vi "Teleop.vi"(10 "Match Info":T2={"Autonomous Elapsed Seconds"=0.0, "TeleOp Elapsed Seconds"=0.0, "Disabled Elapsed Seconds"=0.0, "Visited Autonomous"=FALSE, "Visited TeleOp"=FALSE, "Visited Disabled"=FALSE, "Autonomous Settings"={"Autonomous Style"=enum."Independent", "VI Refnum"=refnum}}, 11 "Call Context":T3) -> ()   [LabVIEW 2016]
doc: "This VI is called for each TeleOp packet received from the DS where the robot is not disabled. It is often used to read from the joysticks and update I/O or to update setpoints for timed control loops. It should complete and return within 20 milliseconds or it may miss DS packets."
uses:
  <vilib>/Rock Robotics/WPI/DriverStation/WPI_DriverStationDerivedRobotMode.ctl
  <vilib>/Rock Robotics/WPI/DriverStation/WPI_DriverStationMatch Info.ctl
  <vilib>/Rock Robotics/WPI/Utilities/WPI_GetSetVariantRefNum.vi
  Robot Global Data.vi
  <vilib>/Rock Robotics/WPI/Solenoid/Deprecated/WPI_SolenoidSetBool.vi
  <vilib>/addons/control/pid/pid.llb/PID (DBL).vi
  navX Library v2/navX Library v2.lvlib
  <vilib>/addons/control/pid/NI_PID_pid.lvlib
panel:
  in  "Mode":bool
  in  "output range":cluster{"output high":dbl, "output low":dbl}={"output high"=100.0, "output low"=-100.0} {"output low" format="%.2f"; "output high" format="%.2f"}
  in  "PID gains":T1={"proportional gain (Kc)"=1.0, "integral time (Ti, min)"=0.01, "derivative time (Td, min)"=0.0} {"derivative time (Td, min)" format="%.3f"; "integral time (Ti, min)" format="%.3f"; "proportional gain (Kc)" format="%.3f"}
  out "Left":dbl(graph)
  out "Right":dbl(graph)
  out "Encoder Right":dbl(graph)
  out "Encoder Left":dbl(graph)
  in  "Speed":dbl=0.5 format="%#_13g"
  out "Out Left":dbl(graph)
  out "Out Right":dbl(graph)
  out "Shooter":cluster{"Sensor Velocity":dbl, dbl, dbl}(graph)
  in  "ShooterRPM":dbl
  in  "P":dbl=0.5 format="%#_13g"
  in  "I":dbl format="%#_13g"
  in  "D":dbl format="%#_13g"
  in  "F":dbl=0.005212 format="%#_13g"
  in  "I Zone":dbl format="%#_13g"
  in  "Ramp Rate":dbl format="%#_13g"
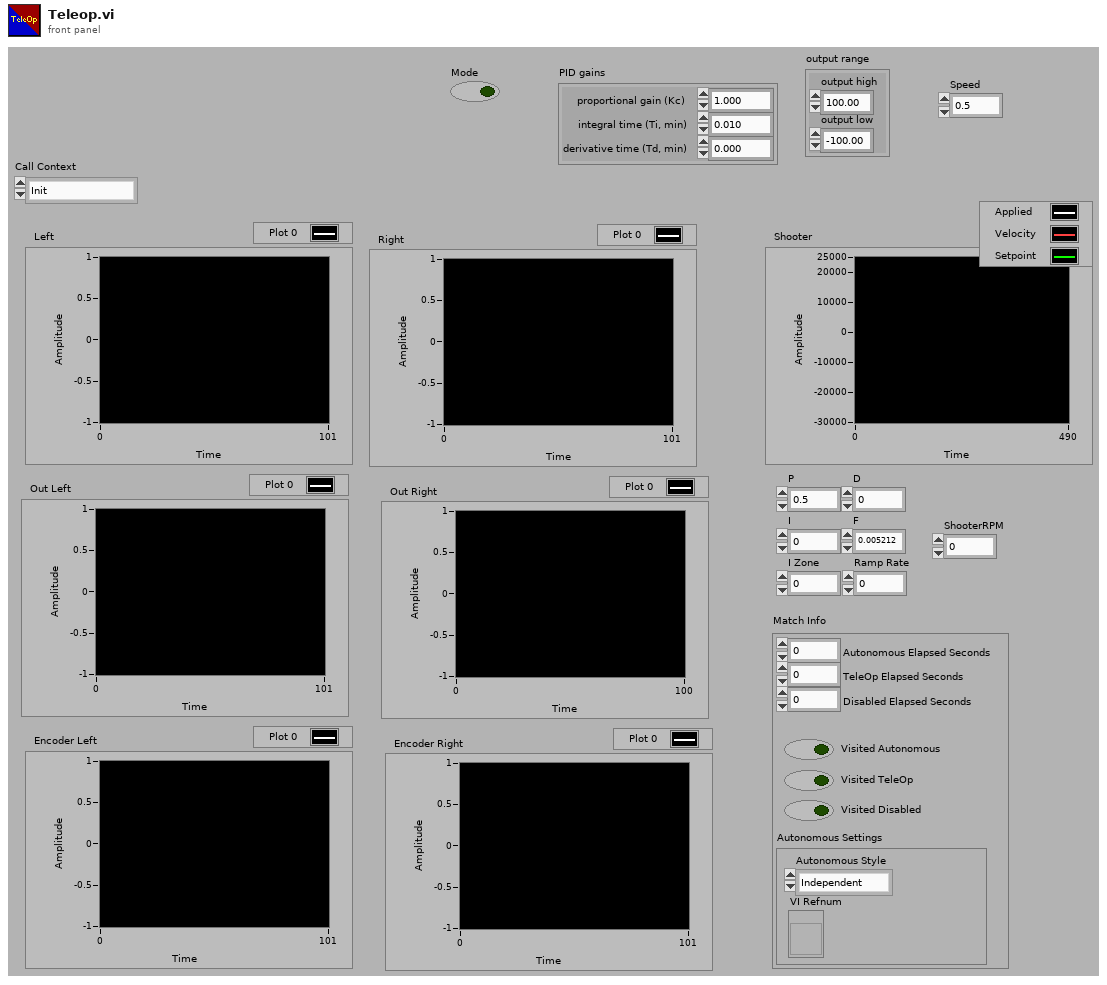
[diagram p1: front panel]
types:
  T1 = cluster{"proportional gain (Kc)":dbl, "integral time (Ti, min)":dbl, "derivative time (Td, min)":dbl}
  T2 = typedef "WPI_DriverStationMatch Info.ctl" = cluster{"Autonomous Elapsed Seconds":dbl, "TeleOp Elapsed Seconds":dbl, "Disabled Elapsed Seconds":dbl, "Visited Autonomous":bool, "Visited TeleOp":bool, "Visited Disabled":bool, "Autonomous Settings":cluster{"Autonomous Style":enum16{"Iterative", "Independent"}, "VI Refnum":refnum<vi>}}
  T3 = typedef "WPI_DriverStationDerivedRobotMode.ctl" = enum16{"Init", "Execute", "Stop"}
  T4 = typedef "WPI_SolenoidDevRef.ctl" = cluster{"DevStatus":errorcluster, "Pneumatics Control Module":u8, "Forward Solenoid Channel":T5, "Reverse Solenoid Channel":T5}
  T5 = typedef "WPI_SolenoidChannel.ctl" = enum8{"Solenoid 0", "Solenoid 1", "Solenoid 2", "Solenoid 3", "Solenoid 4", "Solenoid 5", "Solenoid 6", "Solenoid 7", "Invalid"}
  T6 = typedef "WPI_JoystickDevRef.ctl" = cluster{"Device":T7}
  T7 = typedef "WPI_JoystickDeviceEnum.ctl" = enum16{"USB 0", "USB 1", "USB 2", "USB 3", "USB 4", "USB 5"}
  T8 = cluster{"Buttons[0]":bool, "Buttons[1]":bool, "Buttons[2]":bool, "Buttons[3]":bool, "Buttons[4]":bool, "Buttons[5]":bool, "Buttons[6]":bool, "Buttons[7]":bool, "Buttons[8]":bool}
  T9 = cluster{"Axes[0]":dbl, "Axes[1]":dbl, "Axes[2]":dbl, "Axes[3]":dbl, "Axes[4]":dbl, "Axes[5]":dbl, "Axes[6]":dbl, "Axes[7]":dbl, "Axes[8]":dbl}
  T10 = typedef "navX Library v2.lvlib/Z900_navX_DeviceTypeDef.ctl" = cluster{"Interface":cluster{"Protocol":T11, "Update Rate (4Hz-100Hz)":u8, "navX Open TypeDef":variant}, "Notify Packet":refnum<notifier>, "Loop VI Refnum":refnum<vi>, "Ready to Close Occurrence Refnum":refnum<k4>}
  T11 = typedef "navX Library v2.lvlib/Z900_navX_ProtocolTypeDef.ctl" = enum16{"SERIAL", "I2C", "SPI"}
  T12 = cluster{"Velocity X":dbl, "Velocity Y":dbl, "Velocity Z":dbl, "Displacement X":dbl, "Displacement Y":dbl, "Displacement Z":dbl}
  T13 = cluster{"LinearAcceleration X":dbl, "LinearAcceleration Y":dbl, "LinearAcceleration Z":dbl}
  T14 = cluster{"Quat W":dbl, "Quat X":dbl, "Quat Y":dbl, "Quat Z":dbl}
  T15 = cluster{"Yaw":dbl, "Roll":dbl, "Pitch":dbl, "Heading":dbl, "Fused Heading":dbl}
  T16 = cluster{"Velocity X":dbl, "Velocity Y":dbl, "Velocity Z":dbl, "Displacement X":dbl, "Displacement Y":dbl, "Displacement Z":dbl, "LinearAcceleration X":dbl, "LinearAcceleration Y":dbl, "LinearAcceleration Z":dbl, "Quat W":dbl, "Quat X":dbl, "Quat Y":dbl, "Quat Z":dbl, "Yaw":dbl, "Roll":dbl, "Pitch":dbl}
  T17 = typedef "WPI_MotorControlDeviceRef.ctl" = cluster{"DeviceStatus":errorcluster, "Type":T18, "PWM":cluster{"PWM Channel":T19, "DeadBand":T20}, "CAN":cluster{"Device Number":u8, "SetOutput VI Ref":variant, "GetOutput VI Ref":variant, "Enable VI Ref":variant, "Disable VI Ref":variant, "Data":variant}, "Invert":bool}
  T18 = typedef "WPI_MotorControlType.ctl" = enum16{"PWM", "CAN"}
  T19 = typedef "FPGA_DIOPWMChannel.ctl" = enum8{"PWM 0", "PWM 1", "PWM 2", "PWM 3", "PWM 4", "PWM 5", "PWM 6", "PWM 7", "PWM 8", "PWM 9", "PWM MXP 0", "PWM MXP 1", "PWM MXP 2", "PWM MXP 3", "PWM MXP 4", "PWM MXP 5", "PWM MXP 6", "PWM MXP 7", "PWM MXP 8", "PWM MXP 9", "Invalid"}
  T20 = typedef "WPI_PWMDeadband.ctl" = cluster{"Name":string, "maxPositivePwm":i32, "minPositivePwm":i32, "centerPwm":i32, "maxNegativePwm":i32, "minNegativePwm":i32, "angularRange":u16}
  T21 = typedef "WPI_CANTalonSRX_GlobalStatus.ctl" = cluster{"Applied Throttle":dbl, "Module Enabled":bool, "CAN Error":errorcluster, "Closed Loop Error":dbl, "Forward Limit Switch Closed":bool, "Reverse Limit Switch Closed":bool, "Sensor Position":dbl, "Sensor Velocity":dbl, "Current":dbl, "Sticky Fault - Over Temp":bool, "Sticky Fault - Under Voltage":bool, "Sticky Fault - Forward Limit":bool, "Sticky Fault - Reverse Limit":bool, "Sticky Fault - Forward Soft Limit":bool, "Sticky Fault - Reverse Soft Limit":bool, "Brake is Enabled":bool, "Encoder Position":dbl, "Encoder Velocity":dbl, "Encoder Index Count":dbl, "Encoder A Pin State":bool, "Encoder B Pin State":bool, "Encoder Index Pin State":bool, "Analog In":dbl, "Analog In Velocity":dbl, "Temperature (C)":dbl, "Battery Voltage":dbl, "Control 5 Is Supported":bool, "Current Profile Slot Select":dbl, "Pos Div 8":bool, "Vel Div 4":bool, "Pulse Width Position":i32, "Pulse Width Velocity":i32, "Pulse Width Rise To Rise (us)":i32, "Pulse Width Rise To Fall (us)":i32, "Mot Prof Active Is Under Run":bool, "Mot Prof Active Has Under Run":bool, "Mot Prof Active Is Last":bool, "Mot Prof Active Velocity Only":bool, "Mot Prof Active Is Valid":bool, "Mot Prof Buffer Is Full":bool, "Mot Prof Active Profile Slot Select":i32, "Mot Prof NextID":i32, "Mot Prof Count":i32, "Mot Prof Active Velocity":dbl, "Mot Prof Active Position":dbl, "Mot Prof Output Enable":i32}
  T22 = cluster{dbl, "Sensor Velocity":dbl, "ShooterRPM":dbl}
  T23 = typedef "WPI_RobotDriveDevRef.ctl" = cluster{"DevStatus":errorcluster, "Motors[]":T17[], "Square Inputs":bool, "Max Output":dbl}
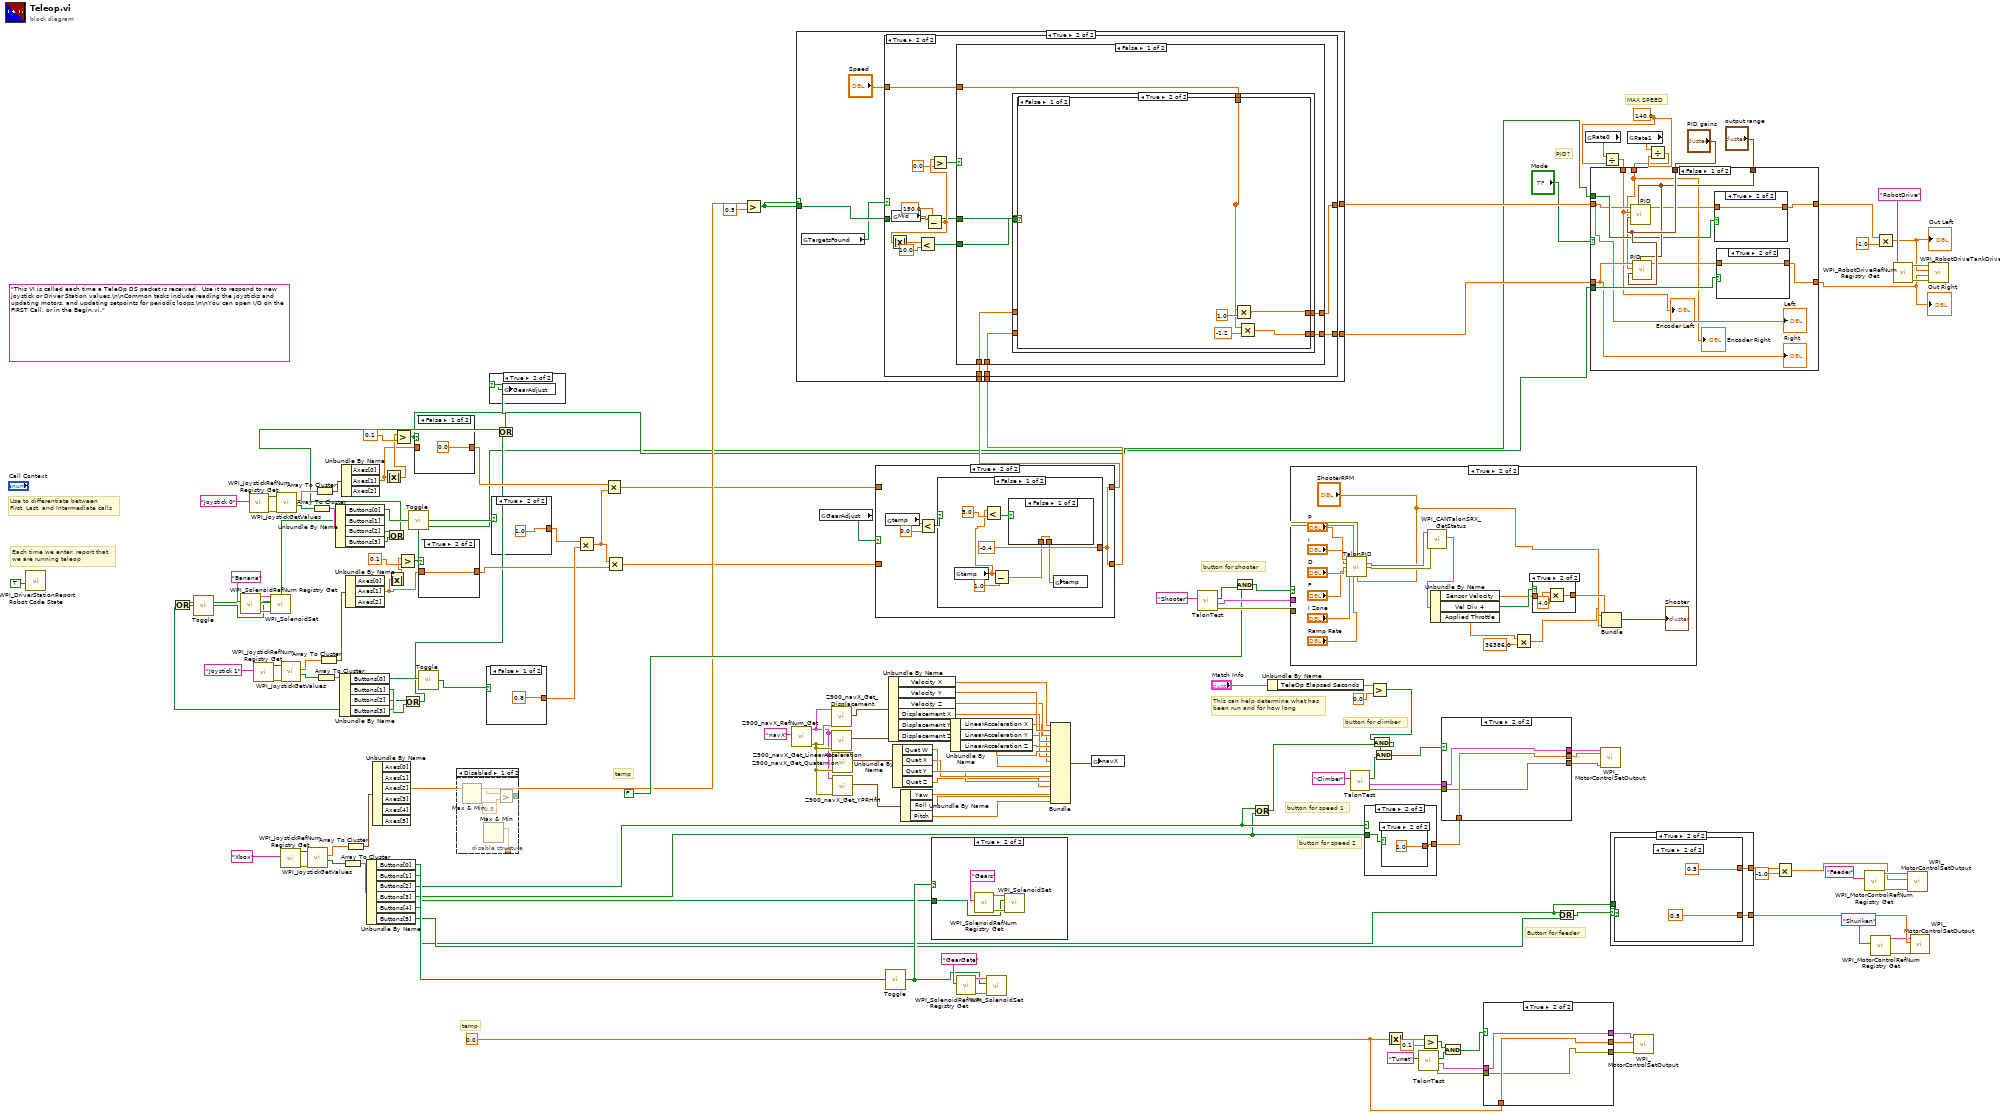
[diagram p0: block diagram]
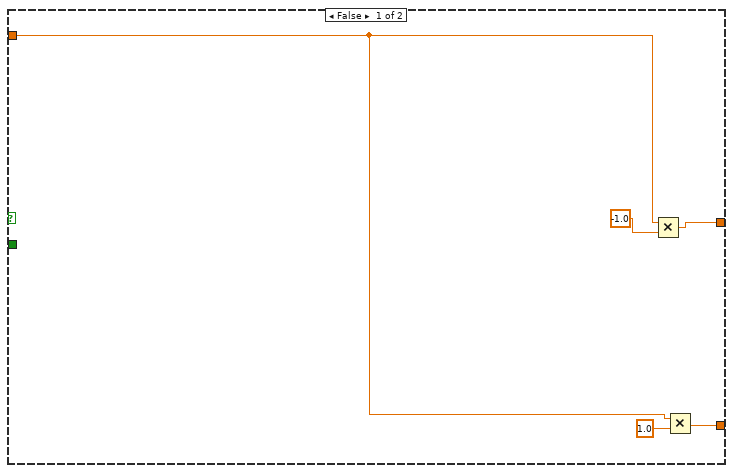
[diagram p3: hidden frame]
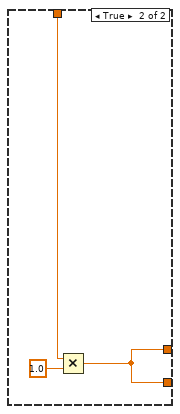
[diagram p5: hidden frame]
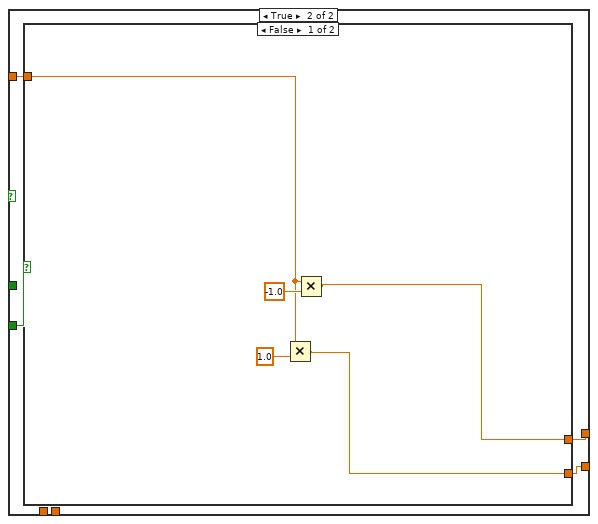
[diagram p6: hidden frame]
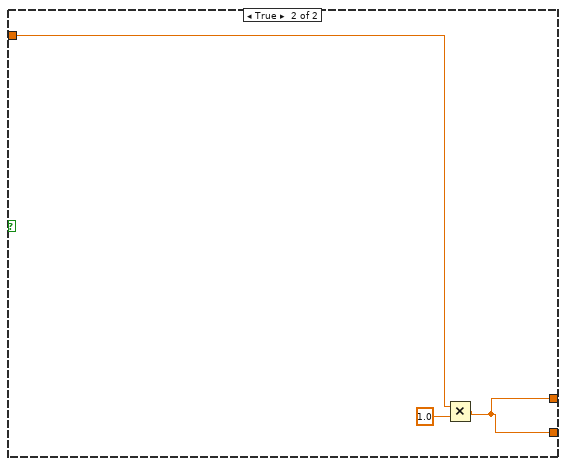
[diagram p7: hidden frame]
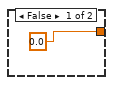
[diagram p8: hidden frame]
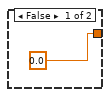
[diagram p9: hidden frame]
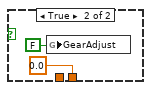
[diagram p14: hidden frame]
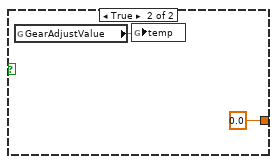
[diagram p15: hidden frame]
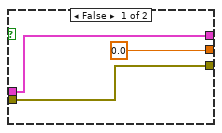
[diagram p16: hidden frame]
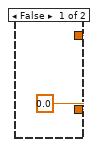
[diagram p18: hidden frame]
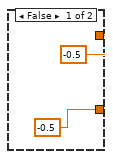
[diagram p19: hidden frame]
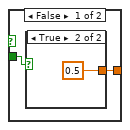
[diagram p20: hidden frame]
diagram:
  w15 = 140.0
  w28 = 0.0
  (unwired) "This VI is called each time a TeleOp DS packet is received.  Use it to respond to new joystick or Driver Station values.\n\nCommon tasks include reading the joysticks and updating motors, and updating setpoints for periodic loops.\n\nYou can open I/O on the FIRST Call, or in the Begin.vi."
  # "MAX SPEED"
  # "PID?"
  # "temp"
  # "temp"
  # "Button for feeder"
  # "button for speed 2"
  # "button for speed 1"
  # "button for climber"
  # "button for shooter"
  # "Each time we enter, report that\nwe are running teleop"
  # "Use to differentiate between\nFirst, Last, and Intermediate calls"
  # "This can help determine what has\nbeen run and for how long"
  n1 = call <vilib>:"WPI_DriverStationReport Robot Code State.vi"("TeleOp"=TRUE ("Autonomous")) -> ()  [unwired: 10 in, 1 out]
  n2 = call <vilib>:"WPI_SolenoidRefNum Registry Get.vi"("refnum name"="Banana") -> ("error out"=w53:errorcluster, "SolenoidDevRef"=w52:T4)  [unwired: 9 in]
  n3 = call <vilib>:"WPI_JoystickRefNum Registry Get.vi"("refnum name"="Joystick 0") -> ("error out"=w155:errorcluster, "JoystickDevRef"=w154:T6)  [unwired: 9 in]
  n4 = call <vilib>:"WPI_JoystickRefNum Registry Get.vi"("refnum name"="Joystick 1") -> ("error out"=w147:errorcluster, "JoystickDevRef"=w146:T6)  [unwired: 9 in]
  n5 = call <vilib>:"WPI_JoystickGetValues.vi"("error in (no error)"=w155, "JoystickDevRef"=w154) -> ("Buttons"=w151:bool[], "Axes"=w152:dbl[])  [unwired: 5 in, 3 out]
  n6 = call <vilib>:"WPI_JoystickRefNum Registry Get.vi"("refnum name"="Xbox") -> ("error out"=w82:errorcluster, "JoystickDevRef"=w81:T6)  [unwired: 9 in]
  n7 = call <vilib>:"WPI_JoystickGetValues.vi"("error in (no error)"=w147, "JoystickDevRef"=w146) -> ("Buttons"=w143:bool[], "Axes"=w144:dbl[])  [unwired: 5 in, 3 out]
  n8 = call <vilib>:"WPI_JoystickGetValues.vi"("error in (no error)"=w82, "JoystickDevRef"=w81) -> ("Buttons"=w78:bool[], "Axes"=w79:dbl[])  [unwired: 5 in, 3 out]
  n9 = Array To Cluster(array=w151) -> (cluster=w149:T8)
  n10 = Array To Cluster(array=w152) -> (cluster=w150:T9)
  n11 = Array To Cluster(array=w143) -> (cluster=w141:T8)
  n12 = Array To Cluster(array=w144) -> (cluster=w142:T9)
  n13 = Unbundle By Name(w149) -> ("Buttons[0]"=w135:bool, "Buttons[1]"=w49:bool, "Buttons[2]"=w34:bool, "Buttons[3]"=w33:bool)
  n14 = Unbundle By Name(w141) -> ("Buttons[0]"=w134:bool, "Buttons[1]"=w48:bool, "Buttons[2]"=w36:bool, "Buttons[3]"=w35:bool)
  n15 = Or(x=w49, y=w48) -> (x .or. y?=w50:bool)
  n16 = call "Toggle.vi"("Input"=w50) -> ("Output"=w47:bool)
  n17 = call-poly <vilib>:"WPI_SolenoidSet.vi"("error in (no error)"=w53, "Value"=w47, "SolenoidDevRef"=w52) -> ()  [unwired: 7 in, 2 out]
  n18 = Unbundle By Name(w150) -> ("Axes[1]"=w136:dbl)  [unwired: 2 out]
  n19 = Array To Cluster(array=w78) -> (cluster=w76:T8)
  n20 = Unbundle By Name(w142) -> ("Axes[1]"=w138:dbl)  [unwired: 2 out]
  n21 = Array To Cluster(array=w79) -> (cluster=w77:T9)
  n22 = Unbundle By Name(w76) -> ("Buttons[0]"=w75:bool, "Buttons[1]"=w74:bool, "Buttons[2]"=w73:bool, "Buttons[3]"=w72:bool, "Buttons[4]"=w69:bool, "Buttons[5]"=w70:bool)
  n23 = Unbundle By Name(w77) -> ("Axes[2]"=w26:dbl)  [unwired: 5 out]
  n24 = Absolute Value(x=w136) -> (abs(x)=w137:dbl)
  n25 = Or(x=w34, y=w33) -> (x .or. y?=w32:bool)
  n26 = Absolute Value(x=w138) -> (abs(x)=w139:dbl)
  n27 = Greater?(x=w137, y=0.1 ("x")) -> (0:w5:bool)
  n28 = Greater?(x=w139, y=0.1 ("x")) -> (0:w4:bool)
  n29 = Or(x=w36, y=w35) -> (x .or. y?=w31:bool)
  n30 = call "Toggle.vi"("Input"=w135) -> ("Output"=w133:bool)
  n31 = case shown="False" w5 {
    tunnel: w136 -> [_ w158]
    tunnel: [0.0 w158] -> w128
    frame False {
    }
    frame True {
    }
  }
  n32 = case shown="True" w4 {
    tunnel: w138 -> [_ w160]
    tunnel: [0.0 w160] -> w129
    frame False {
    }
    frame True {
    }
  }
  n33 = call "Toggle.vi"("Input"=w134) -> ("Output"=w132:bool)
  n34 = disable-structure shown="Disabled" {
    disable-tunnel: [w162 _] -> _
    disable-tunnel: [w161 _] -> _
    frame Disabled {
      n35 = Max & Min() -> (max(x,y)=w164:dbl)  [unwired: 2 in, 1 out]
      n36 = Max & Min() -> (max(x,y)=w161:dbl)  [unwired: 2 in, 1 out]
      n37 = Greater?(x=w164, y=0.5) -> (0:w162:bool)
    }
    frame Enabled {
    }
  }
  n38 = case shown="False" w132 {
    tunnel: [0.8 1.0] -> w130
    frame False {
    }
    frame True {
    }
  }
  n39 = case shown="True" w133 {
    tunnel: [-1.0 1.0] -> w131
    frame False {
    }
    frame True {
    }
  }
  n40 = Or(x=w32, y=w31) -> (x .or. y?=w29:bool)
  n41 = case shown="True" w29 {
    selector: w29 -> [_ w169]
    frame False {
    }
    frame True {
      n42 = global write "Robot Global Data.vi" "GearAdjust"(w169) -> ()
    }
  }
  n43 = Multiply(x=w131, y=w130) -> (x*y=w127:dbl)
  n44 = Multiply(x=w128, y=w127) -> (x*y=w3:dbl)
  n45 = Multiply(x=w127, y=w129) -> (x*y=w2:dbl)
  n46 = Greater?(x=w26, y=0.5) -> (0:w1:bool)
  n47 = call "Z900_navX_RefNum_Get.vi"("refnum name"="navX") -> ("error out"=w125:errorcluster, "navX Device"=w124:T10)  [unwired: 9 in]
  n48 = global read "Robot Global Data.vi" "GearAdjust"() -> (w30:bool)
  n49 = call "Z900_navX_Get_Displacement.vi"("error in (no error)"=w125, "navX Device"=w124) -> ("Displacement"=w120:T12)  [unwired: 6 in, 3 out]
  n50 = call "Z900_navX_Get_LinearAcceleration.vi"("error in (no error)"=w125, "navX Device"=w124) -> ("Linear Acceleration"=w121:T13)  [unwired: 6 in, 3 out]
  n51 = call "Z900_navX_Get_Quaternion.vi"("error in (no error)"=w125, "navX Device"=w124) -> ("Quaternion"=w122:T14)  [unwired: 6 in, 3 out]
  n52 = call "Z900_navX_Get_YPRHfH.vi"("error in (no error)"=w125, "navX Device"=w124) -> ("YRPHfH"=w123:T15)  [unwired: 6 in, 3 out]
  n53 = case shown="True" w30 {
    tunnel: w3 -> [w171 _]
    tunnel: w2 -> [w170 _]
    tunnel: [w171 w172] -> w21
    tunnel: [w170 w172] -> w20
    frame False {
    }
    frame True {
      n54 = global read "Robot Global Data.vi" "temp"() -> (w175:dbl)
      n55 = Less?(x=w175, y=0.0) -> (x < y?=w173:bool)
      n56 = case shown="False" w173 {
        tunnel: [-0.4 0.0] -> w172
        frame False {
          n57 = global read "Robot Global Data.vi" "temp"() -> (w178:dbl)
          n58 = Less?(x=w178, y=5.0 ("x")) -> (x < y?=w179:bool)
          n59 = Subtract(x=w178, y=1.0) -> (x-y=w176:dbl)
          n60 = case shown="False" w179 {
            tunnel: [w183 0.0] -> w177
            tunnel: w176 -> [w183 _]
            frame False {
            }
            frame True {
              n61 = global write "Robot Global Data.vi" "GearAdjust"(FALSE) -> ()
            }
          }
          n62 = global write "Robot Global Data.vi" "temp"(w177) -> ()
        }
        frame True {
          n63 = global read "Robot Global Data.vi" "GearAdjustValue"() -> (w187:dbl)
          n64 = global write "Robot Global Data.vi" "temp"(w187) -> ()
        }
      }
    }
  }
  n65 = case shown="True" w1 {
    tunnel: w21 -> [w189 w196]
    tunnel: w20 -> [w188 w195]
    tunnel: w1 -> [_ w193]
    tunnel: [w189 w192] -> w11
    tunnel: [w188 w191] -> w10
    frame False {
    }
    frame True {
      n66 = global read "Robot Global Data.vi" "TargetsFound"() -> (w190:bool)
      n67 = case shown="True" w190 {
        tunnel: w196 -> [_ w210]
        tunnel: w195 -> [_ w209]
        tunnel: [w199 w208] -> w191
        tunnel: [w200 w207] -> w192
        tunnel: w193 -> [_ w203]
        tunnel: "Speed" -> [w197 w202]
        frame False {
          n68 = Multiply(x=w197, y=-1.0) -> (x*y=w200:dbl)
          n69 = Multiply(x=w197, y=1.0) -> (x*y=w199:dbl)
        }
        frame True {
          n70 = global read "Robot Global Data.vi" "Mid"() -> (w215:dbl)
          n71 = Subtract(x=w215, y=150.0) -> (x-y=w205:dbl)
          n72 = Absolute Value(x=w205) -> (abs(x)=w213:dbl)
          n73 = Less?(x=w213, y=10.0) -> (x < y?=w211:bool)
          n74 = Greater?(x=w205, y=0.0) -> (0:w206:bool)
          n75 = case shown="False" w206 {
            tunnel: w211 -> [w222 w240]
            tunnel: w210 -> [w221 _]
            tunnel: w209 -> [w220 _]
            tunnel: [w219 w238] -> w208
            tunnel: [w218 w239] -> w207
            tunnel: w203 -> [w217 _]
            tunnel: w202 -> [w216 w237]
            frame False {
              n76 = case shown="True" w217 {
                tunnel: w222 -> [_ w228]
                tunnel: w221 -> [w224 _]
                tunnel: w220 -> [w223 _]
                tunnel: [w224 w227] -> w218
                tunnel: [w223 w226] -> w219
                tunnel: w216 -> [_ w225]
                frame False {
                }
                frame True {
                  n77 = case shown="False" w228 {
                    tunnel: [w233 w236] -> w227
                    tunnel: [w231 w236] -> w226
                    tunnel: w225 -> [w229 w234]
                    frame False {
                      n78 = Multiply(x=w229, y=1.0) -> (x*y=w233:dbl)
                      n79 = Multiply(x=w229, y=-1.2) -> (x*y=w231:dbl)
                    }
                    frame True {
                      n80 = Multiply(x=w234, y=1.0) -> (x*y=w236:dbl)
                    }
                  }
                }
              }
            }
            frame True {
              n81 = case shown="False" w240 {
                tunnel: [w245 w248] -> w239
                tunnel: [w243 w248] -> w238
                tunnel: w237 -> [w241 w246]
                frame False {
                  n82 = Multiply(x=w241, y=1.0) -> (x*y=w243:dbl)
                  n83 = Multiply(x=w241, y=-1.0) -> (x*y=w245:dbl)
                }
                frame True {
                  n84 = Multiply(x=w246, y=1.0) -> (x*y=w248:dbl)
                }
              }
            }
          }
        }
      }
    }
  }
  n85 = call "Toggle.vi"("Input"=w75) -> ("Output"=w83:bool)
  n86 = Unbundle By Name(w120) -> ("Velocity X"=w119:dbl, "Velocity Y"=w118:dbl, "Velocity Z"=w117:dbl, "Displacement X"=w116:dbl, "Displacement Y"=w115:dbl, "Displacement Z"=w114:dbl)
  n87 = Unbundle By Name(w122) -> ("Quat W"=w110:dbl, "Quat X"=w109:dbl, "Quat Y"=w108:dbl, "Quat Z"=w107:dbl)
  n88 = Unbundle By Name(w123) -> ("Yaw"=w106:dbl, "Roll"=w105:dbl, "Pitch"=w104:dbl)
  n89 = case shown="True" w83 {
    tunnel: w74 -> [_ w249]
    frame False {
    }
    frame True {
      n90 = call <vilib>:"WPI_SolenoidRefNum Registry Get.vi"("refnum name"="Gears") -> ("error out"=w252:errorcluster, "SolenoidDevRef"=w251:T4)  [unwired: 9 in]
      n91 = call-poly <vilib>:"WPI_SolenoidSet.vi"("error in (no error)"=w252, "Value"=w249, "SolenoidDevRef"=w251) -> ()  [unwired: 7 in, 2 out]
    }
  }
  n92 = Unbundle By Name(w121) -> ("LinearAcceleration X"=w113:dbl, "LinearAcceleration Y"=w112:dbl, "LinearAcceleration Z"=w111:dbl)
  n93 = call <vilib>:"WPI_SolenoidRefNum Registry Get.vi"("refnum name"="GearGate") -> ("error out"=w86:errorcluster, "SolenoidDevRef"=w85:T4)  [unwired: 9 in]
  n94 = call-poly <vilib>:"WPI_SolenoidSet.vi"("error in (no error)"=w86, "Value"=w83, "SolenoidDevRef"=w85) -> ()  [unwired: 7 in, 2 out]
  n95 = Bundle("Velocity X"=w119, "Velocity Y"=w118, "Velocity Z"=w117, "Displacement X"=w116, "Displacement Y"=w115, "Displacement Z"=w114, "LinearAcceleration X"=w113, "LinearAcceleration Y"=w112, "LinearAcceleration Z"=w111, "Quat W"=w110, "Quat X"=w109, "Quat Y"=w108, "Quat Z"=w107, "Yaw"=w106, "Roll"=w105, "Pitch"=w104) -> (w103:T16)  [unwired: 1 in]
  n96 = global write "Robot Global Data.vi" "navX"(w103) -> ()
  n97 = call "TalonTest.vi"("Name"="Shooter") -> ("Output"=w97:bool, "Ref"=w101:T17, "error out"=w100:errorcluster)  [unwired: 7 in]
  n98 = And(x=FALSE, y=w97) -> (x .and. y?=w98:bool)
  n99 = Or(x=w73, y=w72) -> (x .or. y?=w71:bool)
  n100 = Unbundle By Name("Match Info") -> ("TeleOp Elapsed Seconds"=w93:dbl)
  n101 = case shown="True" w98 {
    tunnel: w101 -> [_ w257]
    tunnel: w100 -> [_ w256]
    frame False {
    }
    frame True {
      n102 = call "TalonPID.vi"("P"="P", "Ref In"=w257, "Error in"=w256, "I"="I", "D"="D", "F"="F", "I Zone"="I Zone", "Ramp Rate"="Ramp Rate", "Output"="ShooterRPM") -> ("Ref Out"=w255:T17, "error out"=w254:errorcluster)  [unwired: 5 in]
      n103 = call <vilib>:"WPI_CANTalonSRX_GetStatus.vi"("error in (no error)"=w254, "CAN Talon SRX Ref"=w255) -> ("Talon SRX Status"=w271:T21)  [unwired: 7 in, 2 out]
      n104 = Unbundle By Name(w271) -> ("Sensor Velocity"=w269:dbl, "Vel Div 4"=w270:bool, "Applied Throttle"=w266:dbl)
      n105 = Multiply(x=w266, y=36386.0) -> (x*y=w265:dbl)
      n106 = case shown="True" w270 {
        tunnel: w269 -> [w272 w274]
        tunnel: [w272 w275] -> w264
        frame False {
        }
        frame True {
          n107 = Multiply(x=w274, y=4.0) -> (x*y=w275:dbl)
        }
      }
      n108 = Bundle(w265, "Sensor Velocity"=w264, "ShooterRPM"="ShooterRPM") -> (→"Shooter":T22)  [unwired: 1 in]
    }
  }
  n109 = call "TalonTest.vi"("Name"="Climber") -> ("Output"=w95:bool, "Ref"=w89:T17, "error out"=w88:errorcluster)  [unwired: 7 in]
  n110 = case shown="True" w73 {
    tunnel: [w277 w281] -> w87
    tunnel: w72 -> [w276 w280]
    frame False {
      n111 = case shown="True" w276 {
        tunnel: [0.0 0.5] -> w277
        frame False {
        }
        frame True {
        }
      }
    }
    frame True {
      n112 = case shown="True" w280 {
        tunnel: [0.75 1.0] -> w281
        frame False {
        }
        frame True {
        }
      }
    }
  }
  n113 = Greater?(x=w93, y=0.0) -> (0:w91:bool)
  n114 = And(x=w91, y=w71) -> (x .and. y?=w96:bool)
  n115 = And(x=w96, y=w95) -> (x .and. y?=w90:bool)
  n116 = Absolute Value(x=w28) -> (abs(x)=w62:dbl)
  n117 = call "TalonTest.vi"("Name"="Turret") -> ("Output"=w66:bool, "Ref"=w64:T17, "error out"=w63:errorcluster)  [unwired: 7 in]
  n118 = Greater?(x=w62, y=0.1) -> (0:w60:bool)
  n119 = case shown="True" w90 {
    tunnel: w89 -> [w285 w289]
    tunnel: w88 -> [w284 w287]
    tunnel: w87 -> [_ w288]
    tunnel: [w285 w289] -> w55
    tunnel: [0.0 w288] -> w56
    tunnel: [w284 w287] -> w54
    frame False {
    }
    frame True {
    }
  }
  n120 = And(x=w60, y=w66) -> (x .and. y?=w65:bool)
  n121 = case shown="True" w65 {
    tunnel: w64 -> [w291 w295]
    tunnel: w63 -> [w290 w293]
    tunnel: w28 -> [_ w294]
    tunnel: [w291 w295] -> w59
    tunnel: [0.0 w294] -> w58
    tunnel: [w290 w293] -> w57
    frame False {
    }
    frame True {
    }
  }
  n122 = Or(x=w69, y=w70) -> (x .or. y?=w68:bool)
  n123 = global read "Robot Global Data.vi" "Rate0"() -> (w17:dbl)
  n124 = call <vilib>:"WPI_MotorControlSetOutput.vi"("error in (no error)"=w54, "Output"=w56, "MotorControlDevRef"=w55) -> ()  [unwired: 6 in, 3 out]
  n125 = Divide(x=w17, y=w15) -> (x/y=w14:dbl)
  n126 = case shown="True" w68 {
    tunnel: w69 -> [_ w299]
    tunnel: [w296 w298] -> w39
    tunnel: [w296 w297] -> w46
    frame False {
      w296 = 0.0
    }
    frame True {
      n127 = case shown="True" w299 {
        tunnel: [-0.5 ("Output") 0.5 ("Output")] -> w298
        tunnel: [-0.5 ("Output") 0.5 ("Output")] -> w297
        frame False {
        }
        frame True {
        }
      }
    }
  }
  n128 = global read "Robot Global Data.vi" "Rate1"() -> (w16:dbl)
  n129 = call <vilib>:"WPI_MotorControlSetOutput.vi"("error in (no error)"=w57, "Output"=w58, "MotorControlDevRef"=w59) -> ()  [unwired: 6 in, 3 out]
  n130 = Divide(x=w16, y=w15) -> (x/y=w13:dbl)
  n131 = case shown="False" "Mode" {
    tunnel: w11 -> [w306 w320]
    tunnel: w10 -> [w307 w321]
    tunnel: w14 -> [w305 _]
    tunnel: w13 -> [w304 _]
    tunnel: "PID gains" -> [w315 _]
    tunnel: "output range" -> [w314 _]
    tunnel: w5 -> [w313 _]
    tunnel: w4 -> [w312 _]
    tunnel: [w308 w321] -> w8
    tunnel: [w309 w320] -> w9
    frame False {
      n132 = call-poly <vilib>:"PID.vi"("output range"=w314, "PID gains"=w315, "process variable"=w305, "setpoint"=w306) -> ("output"=w310:dbl)  [unwired: 6 in, 1 out]
      n133 = call-poly <vilib>:"PID.vi"("output range"=w314, "PID gains"=w315, "process variable"=w304, "setpoint"=w307) -> ("output"=w311:dbl)  [unwired: 6 in, 1 out]
      n134 = case shown="True" w313 {
        tunnel: w310 -> [_ w319]
        tunnel: [0.0 w319] -> w309
        frame False {
        }
        frame True {
        }
      }
      n135 = case shown="True" w312 {
        tunnel: w311 -> [_ w317]
        tunnel: [0.0 w317] -> w308
        frame False {
        }
        frame True {
        }
      }
      "Left" <- w306
      "Right" <- w307
      "Encoder Right" <- w304
      "Encoder Left" <- w305
    }
    frame True {
    }
  }
  "Out Right" <- w8
  n136 = Multiply(x=w39, y=-1.0) -> (x*y=w37:dbl)
  n137 = call <vilib>:"WPI_MotorControlRefNum Registry Get.vi"("refnum name"="Feeder") -> ("error out"=w40:errorcluster, "MotorControlDevRef"=w41:T17)  [unwired: 9 in]
  n138 = call <vilib>:"WPI_MotorControlRefNum Registry Get.vi"("refnum name"="Shuriken") -> ("error out"=w42:errorcluster, "MotorControlDevRef"=w43:T17)  [unwired: 9 in]
  n139 = Multiply(x=w9, y=-1.0) -> (x*y=w19:dbl)
  "Out Left" <- w19
  n140 = call <vilib>:"WPI_RobotDriveRefNum Registry Get.vi"("refnum name"="RobotDrive") -> ("error out"=w25:errorcluster, "RobotDriveDevRef"=w24:T23)  [unwired: 9 in]
  n141 = call <vilib>:"WPI_MotorControlSetOutput.vi"("error in (no error)"=w40, "Output"=w37, "MotorControlDevRef"=w41) -> ()  [unwired: 6 in, 3 out]
  n142 = call <vilib>:"WPI_MotorControlSetOutput.vi"("error in (no error)"=w42, "Output"=w46, "MotorControlDevRef"=w43) -> ()  [unwired: 6 in, 3 out]
  n143 = call <vilib>:"WPI_RobotDriveTankDrive.vi"("error in (no error)"=w25, "Right axis value"=w8, "Left axis value"=w19, "RobotDriveDevRef"=w24) -> ()  [unwired: 5 in, 3 out]
